vi "Logic.vi"(8 "error in (no error)":errorcluster, 9 "initialize and close session behavior":T1, 10 "channel list":string, 11 "Session Factory in":refnum<class "Session Factory.lvclass">) -> (0 "error out":errorcluster, 3 "number of samples written per channel":u32)   [LabVIEW 2021, in "DAQmxMeasurement1.lvlib"]
doc: "This VI holds the logic for the NI DAQmx measurement"
uses:
  DAQmxMeasurement1.lvlib
  <vilib>/Plug-In SDKs/Clients/Session Management V1/Session Reservation/Initialize and Close Session Behavior.ctl
  <vilib>/Plug-In SDKs/Sessions/niDAQmx/Session Factory/Session Factory.lvclass
  <vilib>/Plug-In SDKs/Clients/Session Management V1/Session Reservation/Session Reservation.lvclass
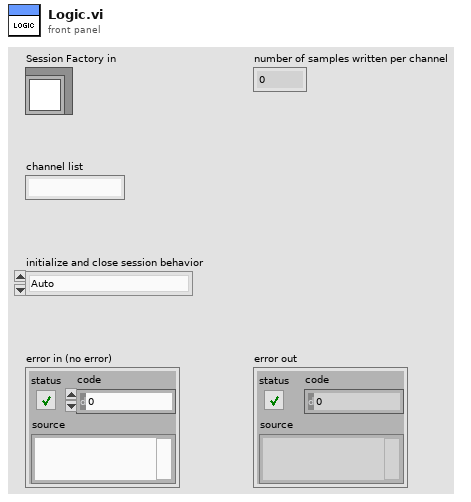
[diagram p1: front panel]
types:
  T1 = typedef "NI Session Management V1 Client.lvlib/Session Reservation.lvclass/Initialize and Close Session Behavior.ctl" = enum16{"Auto", "Initialize and Close", "Attach and Detach", "Initialize and Detach", "Attach and Close"}
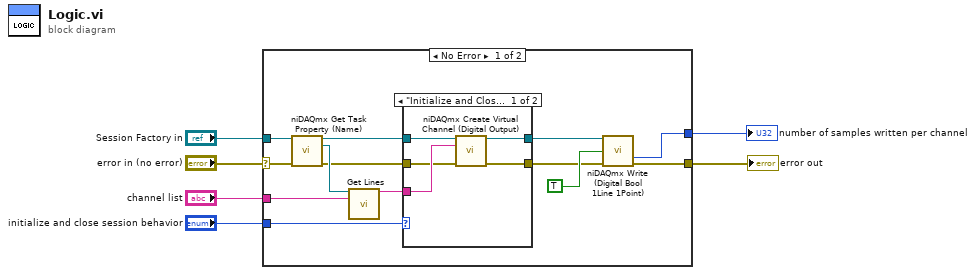
[diagram p0: block diagram]
diagram:
  n1 = case shown="No Error" "error in (no error)" {
    selector: "error in (no error)" -> [w13 w27]
    tunnel: "initialize and close session behavior" -> [w19 _]
    tunnel: "channel list" -> [w18 _]
    tunnel: "Session Factory in" -> [w15 _]
    tunnel: [w12 _] -> w2
    tunnel: [w9 w27] -> w1
    frame No Error {
      n2 = call <vilib>:"niDAQmx Get Task Property (Name).vi"("task in"=w15, "error in"=w13) -> ("task out"=w16:refnum<class "Session Factory.lvclass">, "Name"=w17:refnum<k21>, "error out"=w14:errorcluster)  [unwired: 11 in]
      n3 = call "Get Lines.vi"("task name"=w17, "channel list"=w18) -> ("lines"=w7:tag)  [unwired: 13 in]
      n4 = case shown="\"Initialize and Close\", \"Initialize and Detach\", Default" w19 {
        tunnel: w7 -> [w24 _]
        tunnel: [w23 w25] -> w8
        tunnel: [w22 w26] -> w10
        tunnel: w14 -> [w21 w25]
        tunnel: w16 -> [w20 w26]
        frame "Initialize and Close", "Initialize and Detach", Default {
          n5 = call <vilib>:"niDAQmx Create Virtual Channel (Digital Output).vi"("task in"=w20, "lines"=w24, "error in"=w21) -> ("task out"=w22:refnum<class "Session Factory.lvclass">, "error out"=w23:errorcluster)  [unwired: 11 in]
        }
        frame "Attach and Detach", "Attach and Close" {
        }
      }
      n6 = call <vilib>:"niDAQmx Write (Digital Bool 1Line 1Point).vi"("task in"=w10, "data"=TRUE, "error in"=w8) -> ("number of samples written per channel"=w12:u32, "error out"=w9:errorcluster)  [unwired: 10 in, 1 out]
    }
    frame Error {
    }
  }
  "number of samples written per channel" <- w2
  "error out" <- w1
